vi "FPGA testbench.vi"() -> ()   [LabVIEW 2021]
uses:
  <vilib>/rvi/DesktopExecutionNode/Execution/niFpgaDEN_Execute.vi
  <vilib>/rvi/DesktopExecutionNode/DesktopExecutionNode.xnode
panel:
  in  "stop":bool
  out "Button0":bool
  out "LED3":bool
  out "LED2":bool
  out "LED1":bool
  out "LED0":bool
  out "Pause Led2i":bool
  out "Led1i":bool
  out "Led0i":bool
  out "Led3i":bool
  in  "Count(mSec)":u32
  in  "Pause":bool
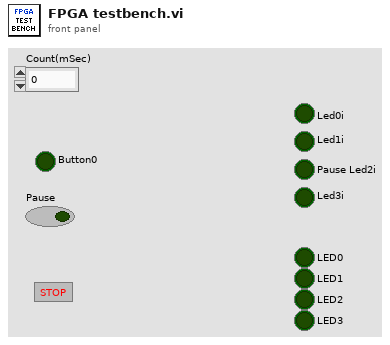
[diagram p1: front panel]
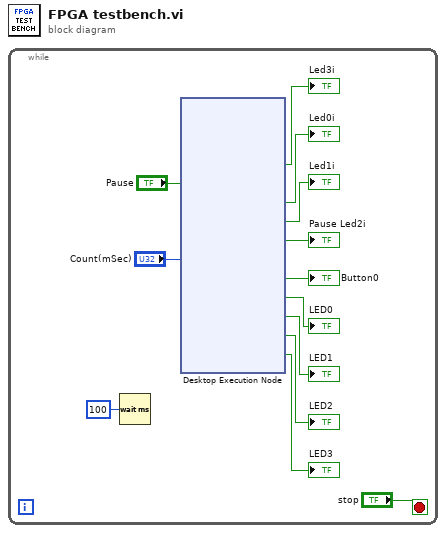
[diagram p0: block diagram]
diagram:
  n1 = while {
    stop <- "stop" stop-if-true
    n2 = Wait (ms)(milliseconds to wait=u32 100) -> ()  [unwired: 1 out]
    n3 = xnode "Desktop Execution Node"("Pause"="Pause", "Count(mSec)"="Count(mSec)") -> ("Led3i"=→"Led3i":bool, "Led0i"=→"Led0i":bool, "Led1i"=→"Led1i":bool, "Pause Led2i"=→"Pause Led2i":bool, "Button0"=→"Button0":bool, "LED0"=→"LED0":bool, "LED1"=→"LED1":bool, "LED2"=→"LED2":bool, "LED3"=→"LED3":bool)  [unwired: 1 in, 1 out]
  }
